vi "Strain measure.vi"(8 "error in":errorcluster caption="에러 입력", 10 "number of samples per channel":i32=1000, 11 "task/channels in":refnum<k21> caption="태스크/채널 입력") -> (0 "error out":errorcluster caption="에러 출력", 2 "data 2":dbl[][](array[numeric]) caption="데이터" format="%0.2f", 3 "task out":refnum<k21> caption="태스크 출력")   [LabVIEW 2013]
uses:
  <vilib>/DAQmx/read.llb/DAQmx Read.vi
  <vilib>/DAQmx/read.llb/DAQmx Read (Analog 2D DBL NChan NSamp).vi
  <vilib>/DAQmx/miscellaneous.llb/DAQmx Fill In Error Info.vi
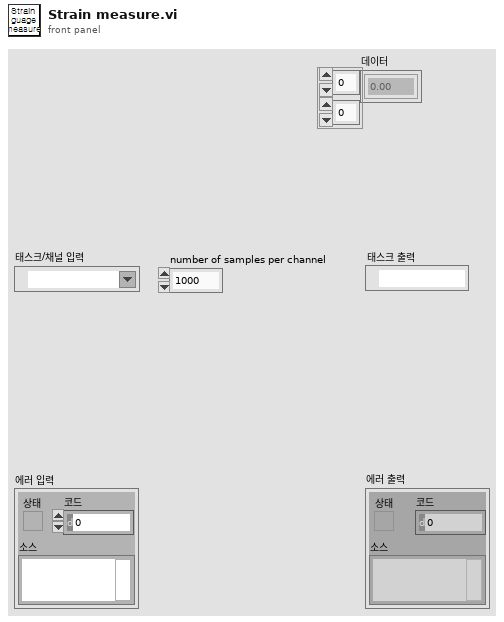
[diagram p1: front panel]
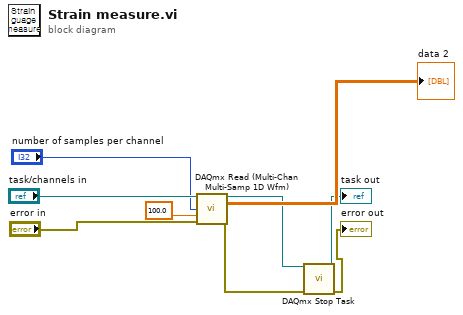
[diagram p0: block diagram]
diagram:
  n1 = call-poly "DAQmx Read (Multi-Chan Multi-Samp 1D Wfm).vi"("task/channels in"="task/channels in", "number of samples per channel"="number of samples per channel", "timeout"=100.0 ("timeout (s)"), "error in"="error in") -> ("task out"=w4:refnum<k21>, "data"=→"data 2":dbl[][], "error out"=w3:errorcluster)  [unwired: 9 in]
  n2 = call <vilib>:"DAQmx Stop Task.vi"("task/channels in"=w4, "error in"=w3) -> ("task out"=→"task out":refnum<k21>, "error out"=→"error out":errorcluster)  [unwired: 12 in]
